vi "Write Admin Data to Report.vi"(8 "error in (no error)":errorcluster, 9 "Cell":string, 10 "text":string, 11 "report in":refnum<class "NI_report.lvclass">) -> (0 "error out":errorcluster, 3 "report out":refnum<class "NI_report.lvclass">)   [LabVIEW 2019]
doc: "For use with Tektronix Excel Data Reports\n\nUsed to write identifying information of the device being tested to the header of the data report."
uses:
  <vilib>/Utility/NIReport.llb/NI_report.lvclass
  <vilib>/addons/_office/_exclsub.llb/font.ctl
  8b1f09da-ba1c-4642-bf12-f9029ae1b83e.vi
  <vilib>/addons/_office/NI_ReportGenerationToolkit.lvlib
  <vilib>/Utility/NIReport.llb/Excel/NI_Excel.lvclass
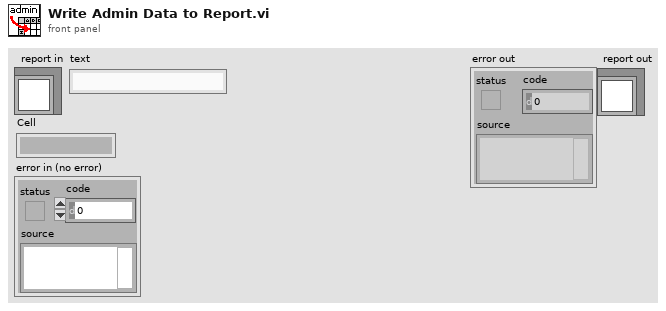
[diagram p1: front panel]
types:
  T1 = typedef "NI_ReportGenerationToolkit.lvlib/font.ctl" = cluster{"font name":string, "font size":dbl, "bold":u16, "italic":u16, "underline":u16, "strike through":u16, "font color":u32}
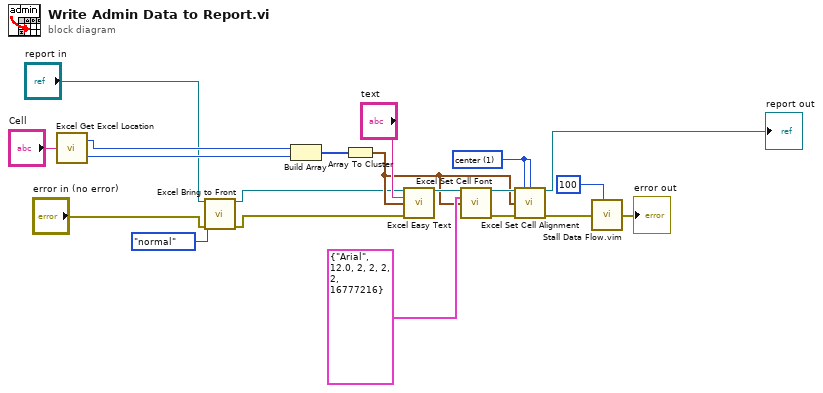
[diagram p0: block diagram]
diagram:
  w13 = 1 items=["left", "center", "right"] ("horizontal alignment (left)")
  n1 = call <vilib>:"Excel Get Excel Location.vi"("cell's name"="Cell") -> ("row"=w19:i32, "column"=w20:i32)
  n2 = call <vilib>:"Excel Bring to Front.vi"("report in"="report in", "window state (maximized)"=enum16{"maximized", "minimized", "normal"}."normal", "error in (no error)"="error in (no error)") -> ("report out"=w2:refnum<class "NI_report.lvclass">, "error out"=w4:errorcluster)  [unwired: 11 in]
  n3 = Build Array(w19, w20) -> (w18:i32[])
  n4 = Array To Cluster(array=w18) -> (cluster=w8:cluster{"[0]":i32, "[1]":i32})
  n5 = call <vilib>:"Excel Easy Text.vi"("report in"=w2, "text"="text", "start (-1, -1)"=w8, "error in (no error)"=w4) -> ("report out"=w11:refnum<class "NI_report.lvclass">)  [unwired: 7 in, 4 out]
  n6 = call <vilib>:"Excel Set Cell Font.vi"("report in"=w11, "font"=T1 {"font name"="Arial", "font size"=12.0, "bold"=2, "italic"=2, "underline"=2, "strike through"=2, "font color"=16777216}, "start (-1, -1)"=w8) -> ("report out"=w12:refnum<class "NI_report.lvclass">, "error out"=w9:errorcluster)  [unwired: 11 in]
  n7 = call <vilib>:"Excel Set Cell Alignment.vi"("report in"=w12, "vertical alignment (top)"=w13, "horizontal alignment (left)"=w13, "start (-1, -1)"=w8, "error in (no error)"=w9) -> ("report out"=→"report out":refnum<class "NI_report.lvclass">, "error out"=w7:errorcluster)  [unwired: 9 in]
  n8 = call "Stall Data Flow.vim"("value in"=w7, "milliseconds to wait"=u32 100) -> ("value out"=→"error out":errorcluster)  [unwired: 1 out]
